vi "subvi_separate.vi"(8 "image data":T1, 9 "subset y":i32, 10 "subset x":i32, 11 "length":i32) -> (3 "separated image array":picture[][](array[picture]))   [LabVIEW 2014]
uses:
  <vilib>/picture/picture.llb/imagedata.ctl
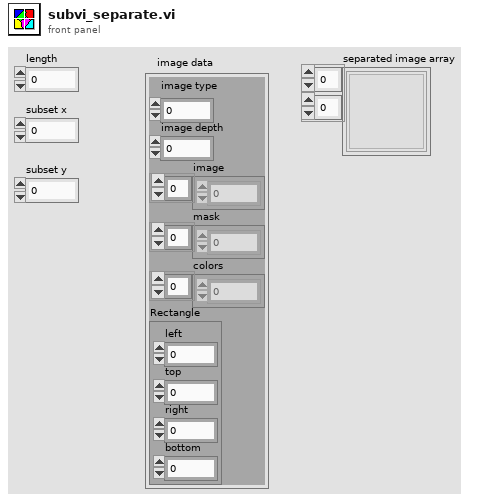
[diagram p1: front panel]
types:
  T1 = typedef "imagedata.ctl" = cluster{"image type":i32, "image depth":i32, "image":u8[], "mask":u8[], "colors":u32[], "Rectangle":cluster{"left":i16, "top":i16, "right":i16, "bottom":i16}}
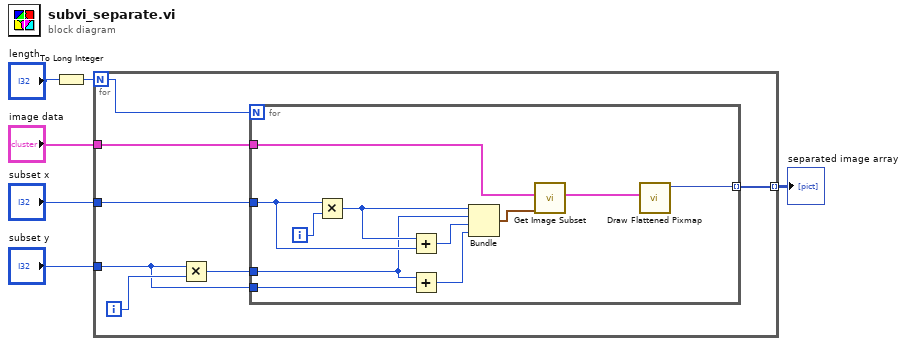
[diagram p0: block diagram]
diagram:
  n1 = To Long Integer(number="length") -> (32bit integer=w5:i32)
  n2 = for {
    N: w5 -> [w11]
    tunnel: "subset x" -> [w8]
    tunnel: "image data" -> [w13]
    tunnel: "subset y" -> [w7]
    tunnel: [w12] -> w1 mode=indexing
    i -> [w10]
    n3 = Multiply(x=w7, y=w10) -> (x*y=w9:i32)
    n4 = for {
      N: w11 -> [_]
      tunnel: w13 -> [w24]
      tunnel: [w22] -> w12 mode=indexing
      tunnel: w9 -> [w16]
      tunnel: w8 -> [w20]
      tunnel: w7 -> [w17]
      i -> [w21]
      n5 = Multiply(x=w20, y=w21) -> (x*y=w19:i32)
      n6 = Add(x=w19, y=w20) -> (x+y=w18:i32)
      n7 = Add(x=w16, y=w17) -> (x+y=w15:i32)
      n8 = Bundle(w19, w16, w18, w15) -> (w14:cluster{i32, i32, i32, i32})  [unwired: 1 in]
      n9 = call <vilib>:"Get Image Subset.vi"("subset rect"=w14, "image data"=w24) -> ("image subset"=w23:T1)  [unwired: 4 in, 1 out]
      n10 = call <vilib>:"Draw Flattened Pixmap.vi"("image data"=w23) -> ("new picture"=w22:picture)  [unwired: 8 in]
    }
  }
  "separated image array" <- w1
